vi "Get FPGA Name From Monkey ID.vi"(8 "error in (no error)":errorcluster, 10 "Monkey ID":string, 11 "Tamer in":refnum<class "Tamer.lvclass">) -> (0 "error out":errorcluster, 2 "FPGA Name":string, 3 "Tamer out":refnum<class "Tamer.lvclass">)   [LabVIEW 2020, in "TALOS.lvlib" / "Tamer.lvlib" / "Tamer.lvclass"]
uses:
  Tamer.lvclass
  Tamer.lvclass/Tamer.ctl
  Ancestor/Ancestor/Ancestor.lvclass/Ancestor.ctl
  FGV/Error Memory/Get Error Description.vi
  Support VIs/Get PC name.vi
  Ancestor/Ancestor/Read ID.vi
  Support VIs/Get Class Name.vi
  <vilib>/Utility/error.llb/Clear Errors.vi
  FGV/Error Memory/Error Memory Core.vi
  <vilib>/AdvancedString/Delimited String to 1D String Array.vi
  Support VIs/Circus Root Path.vi
  FGV/Error Memory/Error Crt Lvl checker.vi
  FGV/Error Memory/Error Memory Core.vi/40c8088d-b597-4017-91af-faa98e00292e.vi
  FGV/Error Memory/Error Memory Core.vi/d4a3ab98-063c-4e44-b43d-fbdcfe6c2be2.vi
  Support VIs/Global Memory.vi
  <vilib>/Utility/LVClass/Get LV Class Name.vi
  Support VIs/Is in Packed Library.vi
  Support VIs/TALOS Root path.vi
  Support VIs/Read CSV worksheet.vi
  Support VIs/Global Constants.vi
  <vilib>/Utility/error.llb/General Error Handler.vi
  Ancestor/Ancestor/Ancestor.lvclass
  <vilib>/Comparison/Equal/Equal Functor/Equal Functor.lvclass
  TALOS.lvlib
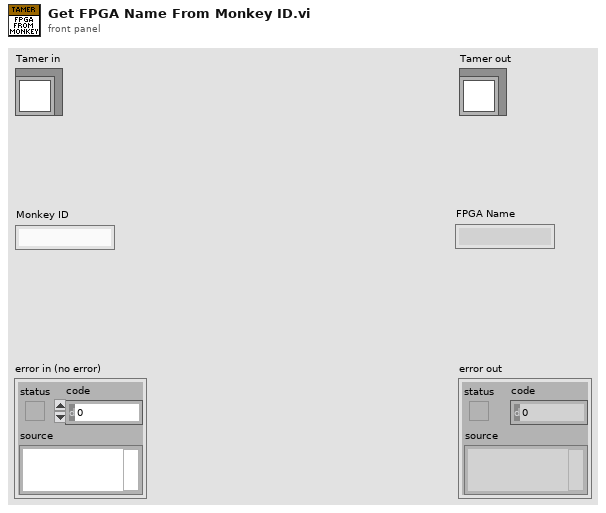
[diagram p1: front panel]
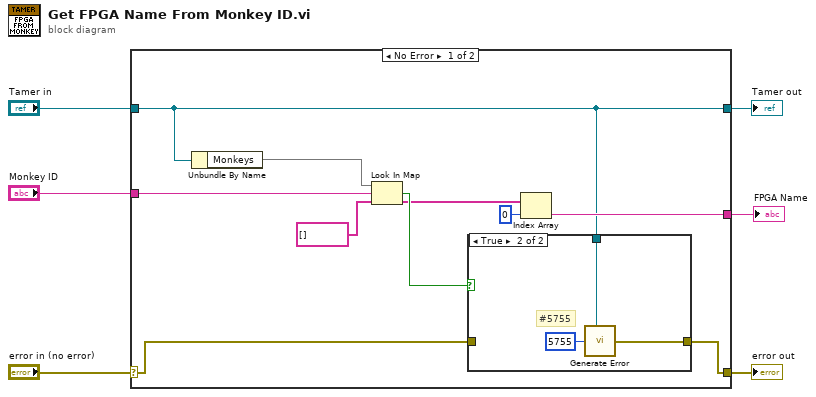
[diagram p0: block diagram]
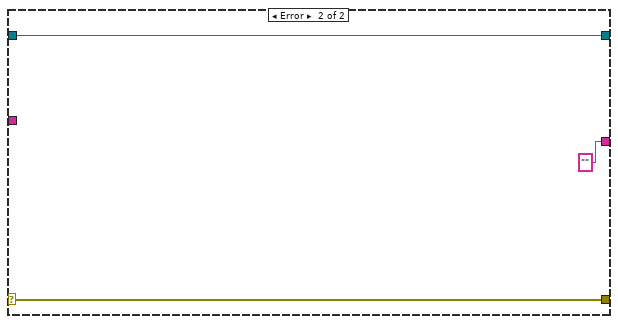
[diagram p3: hidden frame]
diagram:
  n1 = case shown="No Error" "error in (no error)" {
    selector: "error in (no error)" -> [w12 w23]
    tunnel: [w7 w23] -> w5
    tunnel: [w8 w22] -> w3
    tunnel: "Tamer in" -> [w8 w22]
    tunnel: "Monkey ID" -> [w15 _]
    tunnel: [w10 "" ("Kasli Name")] -> w1
    frame No Error {
      n2 = Unbundle By Name(w8) -> ("Monkeys"=w16:map{string, string[]})
      n3 = Look In Map(map=w16, key=w15, default value=string[] []) -> (key not found?=w13:bool, value=w11:string[])
      n4 = case shown="True" w13 {
        tunnel: w12 -> [w17 _]
        tunnel: w8 -> [_ w20]
        tunnel: [w17 w19] -> w7
        frame False {
        }
        frame True {
          # "#5755"
          n5 = call "Generate Error.vi"("Class"=w20, "Error Code"=5755) -> ("error out"=w19:errorcluster)  [unwired: 5 in]
        }
      }
      n6 = Index Array(array=w11, index=0) -> (element=w10:string)
    }
    frame Error {
    }
  }
  "error out" <- w5
  "Tamer out" <- w3
  "FPGA Name" <- w1
